vi "Insert Into Array (Single).vi"(8 "index":i32, 9 "JSON Datatype":refnum<class "JSON Null.lvclass">, 11 "JSON Array in":refnum<class "JSON Array.lvclass">) -> (3 "JSON Array out":refnum<class "JSON Array.lvclass">)   [LabVIEW 2015, in "LVJSON.lvlib" / "JSON Array.lvclass"]
doc: "Inserts an element or subarray into a JSON array at the point you specify in index."
uses:
  JSON Array.lvclass
  JSON Datatype/JSON Null.lvclass
  JSON Array.lvclass/JSON Array.ctl
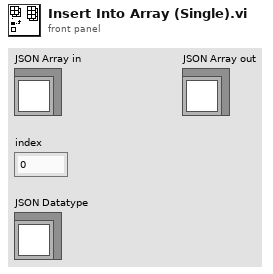
[diagram p1: front panel]
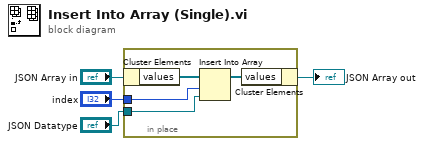
[diagram p0: block diagram]
diagram:
  n1 = in-place {
    in-place-border: "JSON Datatype" -> [w7]
    in-place-border: "index" -> [w8]
    n2 = in-place-cluster #1("JSON Array in") -> ("values"=w6:refnum<class "JSON Null.lvclass">[])
    n3 = Insert Into Array(array=w6, index=w8, new element=w7) -> (w5:refnum<class "JSON Null.lvclass">[])
    n4 = in-place-cluster #1("values"=w5) -> (→"JSON Array out":refnum<class "JSON Array.lvclass">)
  }
